vi "Excess_Water_Temp.vi"() -> (0 "Excess Temp":dbl format="%.2f")   [LabVIEW 2010]
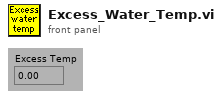
[diagram p1: front panel]
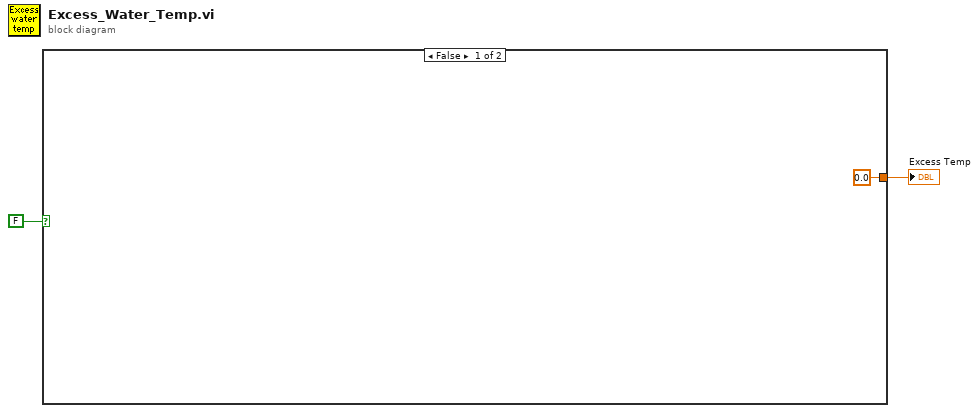
[diagram p0: block diagram]
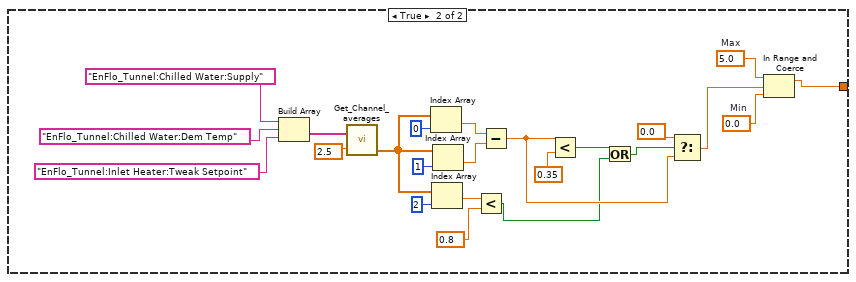
[diagram p2: hidden frame]
diagram:
  n1 = case shown="False" FALSE {
    tunnel: [0.0 ("Max") w4] -> w2
    frame False {
    }
    frame True {
      w16 = 0.0  # Min
      w17 = 5.0  # Max
      n2 = Build Array("EnFlo_Tunnel:Chilled Water:Supply", "EnFlo_Tunnel:Chilled Water:Dem Temp", "EnFlo_Tunnel:Inlet Heater:Tweak Setpoint") -> (w25:string[])
      n3 = call "Get_Channel_averages.vi"("Desired Ch Names"=w25, "Averaging time (mins)"=2.5) -> ("number"=w10:dbl[])  [unwired: 1 in, 2 out]
      n4 = Index Array(array=w10, index=0 ("Index")) -> (element=w20:dbl)
      n5 = Index Array(array=w10, index=2 ("Index")) -> (element=w9:dbl)
      n6 = Index Array(array=w10, index=1 ("Index")) -> (element=w19:dbl)
      n7 = Less?(x=w9, y=0.8) -> (x < y?=w6:bool)
      n8 = Subtract(x=w20, y=w19) -> (x-y=w15:dbl)
      n9 = Less?(x=w15, y=0.35) -> (x < y?=w7:bool)
      n10 = Or(x=w7, y=w6) -> (x .or. y?=w5:bool)
      n11 = Select(t=0.0, s=w5, f=w15) -> (s? t:f=w13:dbl)
      n12 = In Range and Coerce(upper limit=w17, x=w13, lower limit=w16) -> (coerced(x)=w4:dbl)  [unwired: 1 out]
    }
  }
  "Excess Temp" <- w2
